vi "Current Channels Array.vi"(8 "error in":errorcluster, 11 "Channel 1":string) -> (0 "error out":errorcluster, 1 "Current Channel?":bool, 2 "Channel 2":string, 3 "Channel 1":string)   [LabVIEW 2021, in "DMM_Scan PXI Mux PXI Shunt 16V-15C.lvlib"]
doc: "Checks if the channel is a current channel (16 to 30) and provide chX comX names for individual relay paths.\n\nReturns True if Channel 1 part of a current channel mapping."
uses:
  DMM_Scan PXI Mux PXI Shunt 16V-15C.lvlib
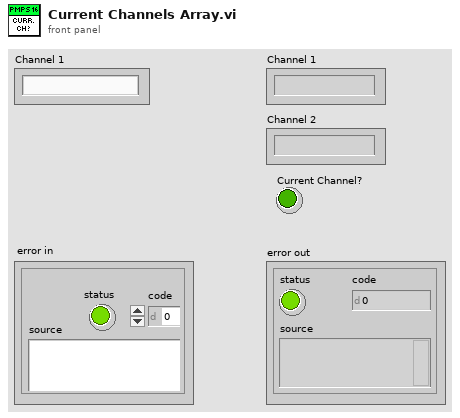
[diagram p1: front panel]
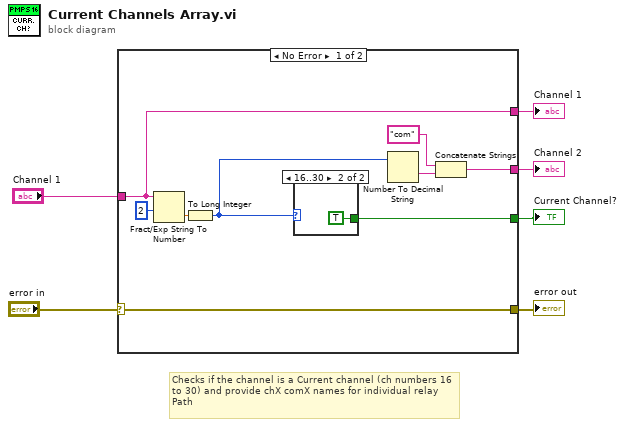
[diagram p0: block diagram]
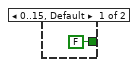
[diagram p2: hidden frame]
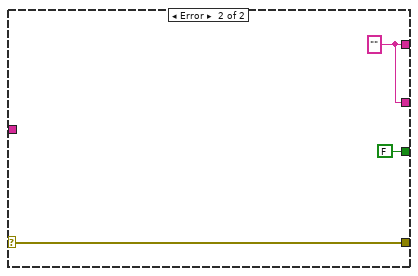
[diagram p3: hidden frame]
diagram:
  # "Checks if the channel is a Current channel (ch numbers 16 to 30) and provide chX comX names for individual relay Path"
  n1 = case shown="No Error" "error in" {
    selector: "error in" -> [w13 w20]
    tunnel: "Channel 1" -> [w7 _]
    tunnel: [w13 w20] -> w4
    tunnel: [w12 FALSE] -> w3
    tunnel: [w8 w18] -> w2
    tunnel: [w7 w18] -> w1
    frame No Error {
      n2 = Fract/Exp String To Number(string=w7, offset=2 ("offset (0)")) -> (number=w14:dbl)  [unwired: 2 in, 1 out]
      n3 = To Long Integer(number=w14) -> (32bit integer=w9:i32)
      n4 = case shown="16..30" w9 {
        tunnel: [FALSE TRUE] -> w12
        frame 0..15, Default {
        }
        frame 16..30 {
        }
      }
      n5 = Number To Decimal String(number=w9) -> (decimal integer string=w11:string)  [unwired: 1 in]
      n6 = Concatenate Strings("com", w11) -> (w8:string)
    }
    frame Error {
      w18 = ""
    }
  }
  "error out" <- w4
  "Current Channel?" <- w3
  "Channel 2" <- w2
  "Channel 1" <- w1
